vi "ApplyVIPC--function.vi"(8 "error in":errorcluster, 10 "Timeout in seconds":dbl=60.0, 11 "VIPC File Path":path) -> (0 "error out":errorcluster, 2 "Need to Apply?":bool)   [LabVIEW 2020, in "CICD.lvlib"]
doc: "Apply VI Package Configuration (.vipc file).\nThis VI applys the VIPC to the LabVIEW IDE."
uses:
  CICD.lvlib
  <vilib>/JKI/VIPM API/VIPM API_vipm_api.lvlib
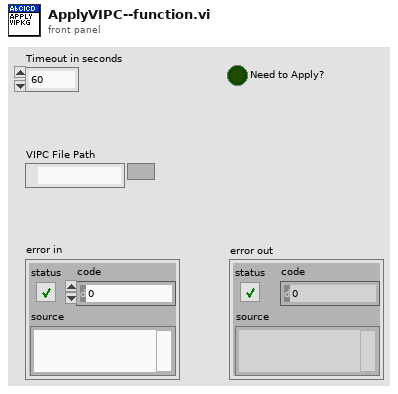
[diagram p1: front panel]
types:
  T1 = typedef "VIPM API_vipm_api.lvlib/LabVIEW Target Info Cluster_vipm_api.ctl" = cluster{"Version":string, "Connection Tested":bool, "Disabled":bool}
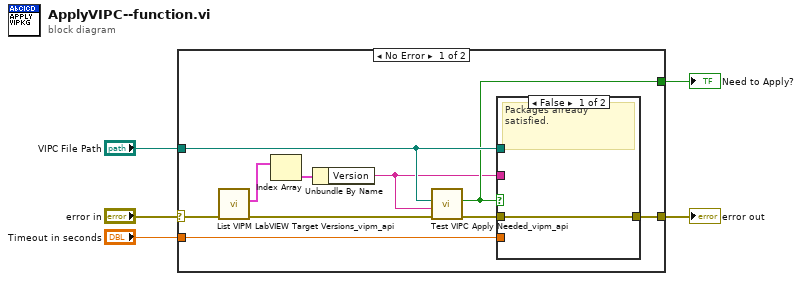
[diagram p0: block diagram]
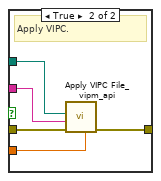
[diagram p2: hidden frame]
diagram:
  n1 = case shown="No Error" "error in" {
    selector: "error in" -> [w12 w22]
    tunnel: [w13 w22] -> w5
    tunnel: "Timeout in seconds" -> [w11 _]
    tunnel: "VIPC File Path" -> [w8 _]
    tunnel: [w7 _] -> w1
    frame No Error {
      n2 = call <vilib>:"List VIPM LabVIEW Target Versions_vipm_api.vi"("error in (no error)"=w12) -> ("error out"=w15:errorcluster, "LabVIEW Target Info"=w9:T1[])  [unwired: 9 in]
      n3 = Index Array(array=w9) -> (element=w10:T1)  [unwired: 1 in]
      n4 = Unbundle By Name(w10) -> ("Version"=w6:string)
      n5 = call <vilib>:"Test VIPC Apply Needed_vipm_api.vi"("error in (no error)"=w15, "LabVIEW Version (use vipc version)"=w6, "VIPC File Path"=w8) -> ("error out"=w14:errorcluster, "Need to Apply?"=w7:bool)  [unwired: 6 in, 1 out]
      n6 = case shown="False" w7 {
        tunnel: w14 -> [w16 w21]
        tunnel: [w16 w20] -> w13
        tunnel: w8 -> [_ w19]
        tunnel: w11 -> [_ w18]
        tunnel: w6 -> [_ w17]
        frame False {
          # "Packages already satisfied."
        }
        frame True {
          # "Apply VIPC."
          n7 = call <vilib>:"Apply VIPC File_vipm_api.vi"("Timeout in seconds (0: no timeout)"=w18, "error in (no error)"=w21, "LabVIEW Version"=w17, "VIPC File"=w19) -> ("error out"=w20:errorcluster)  [unwired: 7 in]
        }
      }
    }
    frame Error {
    }
  }
  "error out" <- w5
  "Need to Apply?" <- w1
